vi "subGetDependentLibsFromLinker.vi"(9 "Name":string, 11 "Path":path) -> (3 "Dependent libs":string[](array[string]))   [LabVIEW 2020, in "SolutionBuilder.lvlib" / "SolutionBuilder.lvclass"]
uses:
  SolutionBuilder.lvclass
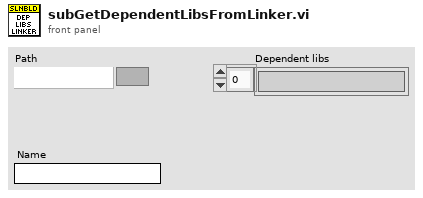
[diagram p1: front panel]
types:
  T1 = typedef "NI_FileType.lvlib/LVFileType.ctl" = enum32{"Invalid file", "Unknown type", "Instrument", "Control", "Polymorphic VI", "Project", "Library", "LVClass", "XControl", "XNode", "Shared library", ".NET assembly", "ActiveX interface", "CIN", "Run-time menu", "Palette menu", "Help file", "LLB", "XNode Edit Dependency", "Class Private Data Control", "Statechart", "MathScript .m file", "Ladder Diagram", "LVLibp", "XNode Build Dependency"}
  T2 = cluster{"path":path, "delimited name":string, "type":T1, "iState":u32, "iStyle":u16, "wStyle":u16, "buttons":u16, "viflags":u32, "viflags2":u32, "links":u32[]}[]
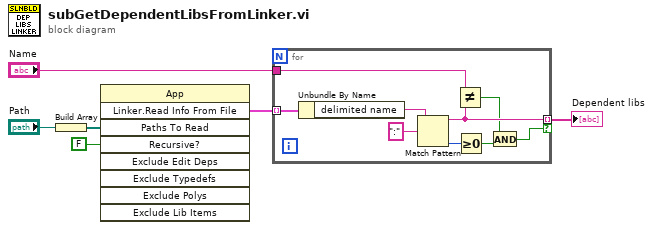
[diagram p0: block diagram]
diagram:
  n1 = Build Array("Path") -> (w3:path[])
  n2 = invoke class="App" method="Linker.Read Info From File"("Paths To Read"=w3, "Recursive?"=FALSE) -> ("Linker.Read Info From File"=w4:T2)  [unwired: 7 in, 8 out]
  n3 = for {
    tunnel: w4 -> [w15] mode=indexing
    tunnel: [w10] -> w5 mode=indexing if=w7
    tunnel: "Name" -> [w11]
    n4 = Unbundle By Name(w15) -> ("delimited name"=w13:string)
    n5 = Match Pattern(string=w13, regular expression=":") -> (before substring=w10:string, offset past match=w12:i32)  [unwired: 1 in, 2 out]
    n6 = Not Equal?(x=w11, y=w10) -> (x != y?=w9:bool)
    n7 = Greater Or Equal To 0?(x=w12) -> (x >= 0?=w8:bool)
    n8 = And(x=w9, y=w8) -> (x .and. y?=w7:bool)
  }
  "Dependent libs" <- w5
